vi "Actors Test.vi"() -> ()   [LabVIEW 2020, in "RTAF.lvlib"]
uses:
  RTAF.lvlib
  Test/Actor/Count Behaviour.ctl
  Logger/Actor/Config.ctl
  Alarms Handler/Actor/Config.ctl
  Logger/API/Logger Actor API.lvclass
  C:/dev/PGS/2001 - TBCM/Source/RT/RTAF/Source/RTAF/Actors/Base Actor/API/Actor API.lvclass
  Test/API/Test Actor API.lvclass
  Alarms Handler/API/Alarms Handler Actor API.lvclass
  Global References.vi
  Base Actor/API/Actor API.lvclass
  Logger/Actor/Logger Actor.lvclass
  C:/dev/PGS/2001 - TBCM/Source/RT/RTAF/Source/RTAF/Actors/Logger/API/Logger Actor API.lvclass
  Test/Actor/Test Actor.lvclass
  C:/dev/PGS/2001 - TBCM/Source/RT/RTAF/Source/RTAF/Actors/Test/API/Test Actor API.lvclass
  Alarms Handler/Actor/Alarms Handler Actor.lvclass
  C:/dev/PGS/2001 - TBCM/Source/RT/RTAF/Source/RTAF/Actors/Alarms Handler/API/Alarms Handler Actor API.lvclass
  System Status/API/System Status Actor API.lvclass
  System Status/Actor/System Status Actor.lvclass
  C:/dev/PGS/2001 - TBCM/Source/RT/RTAF/Source/RTAF/Actors/System Status/API/System Status Actor API.lvclass
  System Status/Actor/Total Used Free MB.ctl
panel:
  out "Uptime":dbl format="%<%H:%M:%S%1u>t"
  out "Disk":T1
  out "Memory":T1
  in  "error in":errorcluster
  in  "Add Alarm":bool
  in  "Test Window State":T2(ring)
  in  "Alarm":string
  in  "Add Alarm":bool
  in  "Log Status":bool
  in  "Status":string
  in  "Alarms Handler Window State":T2(ring)
  in  "Logger Window State":T2(ring)
  out "Test Count":i32
  in  "Get Test Count":bool
  in  "Test Count Behaviour":T3
  # "Test"
  # "Logger"
  # "Alarms"
  # "System Status"
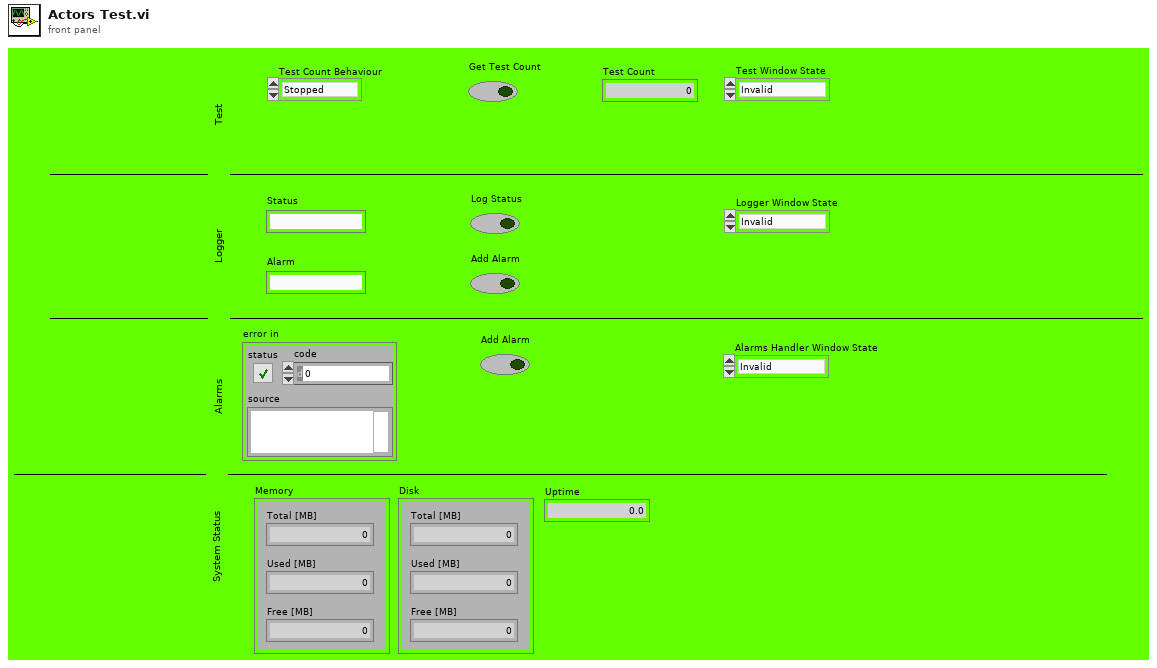
[diagram p1: front panel]
types:
  T1 = typedef "RTAF.lvlib/System Status Actor.lvclass/Total Used Free MB.ctl" = cluster{"Total [MB]":dbl, "Used [MB]":dbl, "Free [MB]":dbl}
  T2 = enum32{"Invalid", "Standard", "Closed", "Hidden", "Minimized", "Maximized"}
  T3 = typedef "RTAF.lvlib/Test Actor.lvclass/Count Behaviour.ctl" = enum16{"Stopped", "Up", "Down"}
  T4 = typedef "RTAF.lvlib/Alarms Handler Actor.lvclass/Config.ctl" = cluster{"Max Alarms Before Reset":i32}
  T5 = typedef "RTAF.lvlib/Logger Actor.lvclass/Config.ctl" = cluster{"Log Files Directory":path, "Max Lines Per File":i32}
  T6 = cluster{"System Status Actor":refnum<event-registration>}
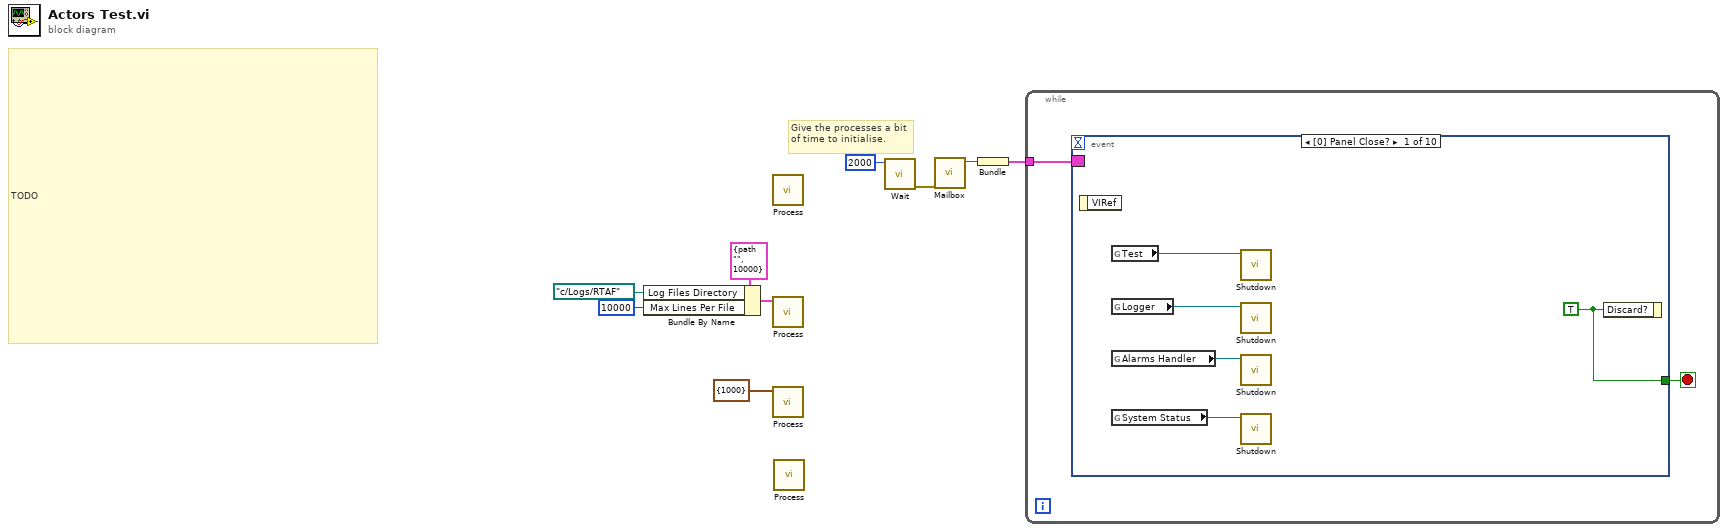
[diagram p0: block diagram]
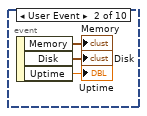
[diagram p2: hidden frame]
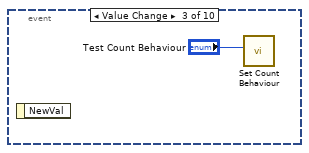
[diagram p3: hidden frame]
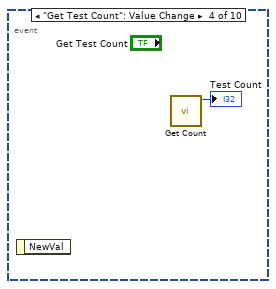
[diagram p4: hidden frame]
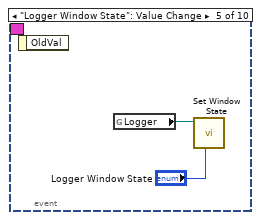
[diagram p5: hidden frame]
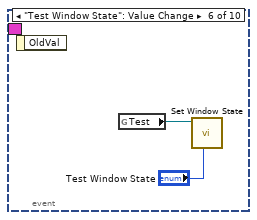
[diagram p6: hidden frame]
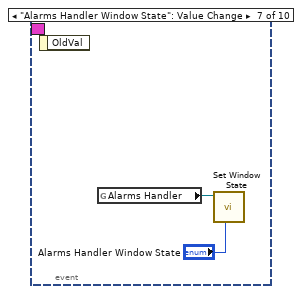
[diagram p7: hidden frame]
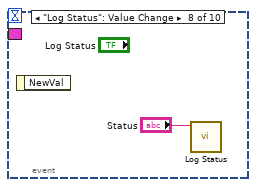
[diagram p8: hidden frame]
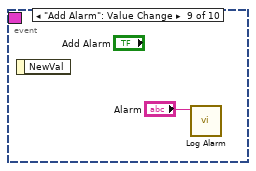
[diagram p9: hidden frame]
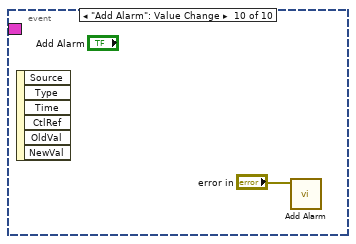
[diagram p10: hidden frame]
diagram:
  # "Give the processes a bit of time to initialise."
  # "TODO"
  n1 = Bundle By Name(cluster=T5 {"Log Files Directory"=path "", "Max Lines Per File"=10000} ("Initial Config"), "Log Files Directory"=path "c:/Logs/RTAF", "Max Lines Per File"=10000) -> (w8:T5)
  n2 = call "Process.vi"() -> ()  [unwired: 12 in]
  n3 = call "Process.vi"("Initial Config"=w8) -> ()  [unwired: 11 in]
  n4 = call "Process.vi"("Config"=T4 {"Max Alarms Before Reset"=1000}) -> ()  [unwired: 11 in]
  n5 = call "Process.vi"() -> ()  [unwired: 12 in]
  n6 = call "Wait.vi"("Wait Time [ms]"=u32 2000) -> ("error out"=w4:errorcluster)  [unwired: 10 in]
  n7 = call "Mailbox.vi"("error in (no error)"=w4) -> ("System Status Actor"=w3:refnum<event-registration>)  [unwired: 9 in, 1 out]
  n8 = Bundle("System Status Actor"=w3) -> (w2:T6)  [unwired: 1 in]
  n9 = while {
    tunnel: w2 -> [w10]
    stop <- w11 stop-if-true
    n10 = event shown="[0] Panel Close?" {
      selector: w10 -> [_ _ _ _ _ _ _ _ _ _]
      dyn-events: _ -> [_ _ _ _ _ _ _ _ _ _]
      timeout: _ -> [_ _ _ _ _ _ _ _ _ _]
      tunnel: [w16 _ _ _ _ _ _ _ _ _] -> w11
      event Panel Close? {
        w16 = TRUE ("Discard?")
        n11 = event-data() -> ()  [unwired: 1 in, 1 out]
        n12 = global read "Global References.vi" "Test"() -> (w14:refnum<class "Test Actor API.lvclass">)
        n13 = global read "Global References.vi" "Logger"() -> (w15:refnum<class "Logger Actor API.lvclass">)
        n14 = global read "Global References.vi" "Alarms Handler"() -> (w13:refnum<class "Alarms Handler Actor API.lvclass">)
        n15 = global read "Global References.vi" "System Status"() -> (w12:refnum<class "System Status Actor API.lvclass">)
        n16 = call "Shutdown.vi"("Actor API"=w14) -> ()  [unwired: 10 in, 1 out]
        n17 = call "Shutdown.vi"("Actor API"=w15) -> ()  [unwired: 10 in, 1 out]
        n18 = call "Shutdown.vi"("Actor API"=w13) -> ()  [unwired: 10 in, 1 out]
        n19 = call "Shutdown.vi"("Actor API"=w12) -> ()  [unwired: 10 in, 1 out]
        n20 = event-data("Discard?"=w16) -> ()  [unwired: 1 in, 1 out]
      }
      event User Event {
        n21 = event-data() -> ("Memory"=→"Memory":T1, "Disk"=→"Disk":T1, "Uptime"=→"Uptime":dbl)  [unwired: 1 in]
      }
      event Value Change {
        n22 = event-data() -> ()  [unwired: 1 in, 1 out]
        n23 = call "Set Count Behaviour.vi"("Count Behaviour"="Test Count Behaviour") -> ()  [unwired: 10 in, 1 out]
      }
      event "Get Test Count": Value Change {
        n24 = event-data() -> ()  [unwired: 1 in, 1 out]
        n25 = call "Get Count.vi"() -> ("Count"=→"Test Count":i32)  [unwired: 10 in, 1 out]
      }
      event "Logger Window State": Value Change {
        n26 = event-data() -> ()  [unwired: 1 in, 1 out]
        n27 = global read "Global References.vi" "Logger"() -> (w22:refnum<class "Logger Actor API.lvclass">)
        n28 = call "Set Window State.vi"("State"="Logger Window State", "Actor API"=w22) -> ()  [unwired: 9 in, 1 out]
      }
      event "Test Window State": Value Change {
        n29 = event-data() -> ()  [unwired: 1 in, 1 out]
        n30 = global read "Global References.vi" "Test"() -> (w25:refnum<class "Test Actor API.lvclass">)
        n31 = call "Set Window State.vi"("State"="Test Window State", "Actor API"=w25) -> ()  [unwired: 9 in, 1 out]
      }
      event "Alarms Handler Window State": Value Change {
        n32 = event-data() -> ()  [unwired: 1 in, 1 out]
        n33 = global read "Global References.vi" "Alarms Handler"() -> (w26:refnum<class "Alarms Handler Actor API.lvclass">)
        n34 = call "Set Window State.vi"("State"="Alarms Handler Window State", "Actor API"=w26) -> ()  [unwired: 9 in, 1 out]
      }
      event "Log Status": Value Change {
        n35 = event-data() -> ()  [unwired: 1 in, 1 out]
        n36 = call "Log Status.vi"("Message"="Status") -> ()  [unwired: 10 in, 1 out]
      }
      event "Add Alarm": Value Change {
        n37 = event-data() -> ()  [unwired: 1 in, 1 out]
        n38 = call "Log Alarm.vi"("Message"="Alarm") -> ()  [unwired: 10 in, 1 out]
      }
      event "Add Alarm": Value Change {
        n39 = event-data() -> ()  [unwired: 1 in, 6 out]
        n40 = call "Add Alarm.vi"("Alarm"="error in") -> ()  [unwired: 10 in, 1 out]
      }
    }
  }
